vi "Agilent VNA Filter Unmeasurable Measurements.vi"(7 "Agilent VNA":T5, 8 "error in (no error)":errorcluster, 10 "Parameters to Measure":T1[](array[typedef]) {"Channel" min=1 max=99 step=1; "Parameter"."Stimulus Port" min=1 step=1; "Parameter"."Response Port" min=1 step=1}, 11 "VISA Resource Name":refnum<visa-resource-name>) -> (0 "error out":errorcluster, 1 "Removed Parameters":T1[](array[typedef]) {"Channel" min=1 max=99 step=1; "Parameter"."Stimulus Port" min=1 step=1; "Parameter"."Response Port" min=1 step=1}, 2 "Filtered Parameters to Measure":T1[](array[typedef]) {"Channel" min=1 max=99 step=1; "Parameter"."Stimulus Port" min=1 step=1; "Parameter"."Response Port" min=1 step=1}, 3 "dup VISA Resource Name":refnum<visa-resource-name>, 4 "Measurements Removed?":bool)   [LabVIEW 2011]
uses:
  tests/S Parameter/TypeDefs/SP Parameter to Measure.ctl
  tests/S Parameter/TypeDefs/SP Parameter.ctl
  tests/S Parameter/TypeDefs/SP Calibration State.ctl
  tests/S Parameter/TypeDefs/SP Measurement Format.ctl
  TypeDefs/Agilent VNA Instrument Info.ctl
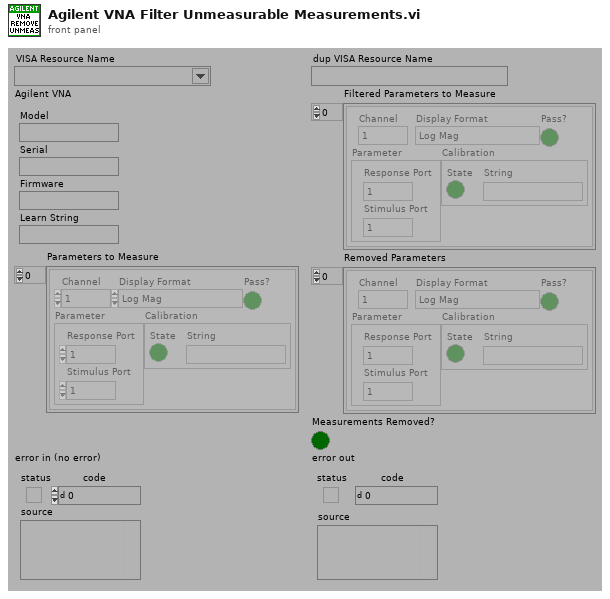
[diagram p1: front panel]
types:
  T1 = typedef "SP Parameter to Measure.ctl" = cluster{"Channel":i8, "Parameter":T2, "Calibration":T3, "Display Format":T4, "Pass?":bool}
  T2 = typedef "SP Parameter.ctl" = cluster{"Stimulus Port":i8, "Response Port":i8}
  T3 = typedef "SP Calibration State.ctl" = cluster{"State":bool, "String":string}
  T4 = typedef "SP Measurement Format.ctl" = enum32{"Log Mag", "Phase", "Delay", "Smith (R+jX)", "Polar (Re/Im)", "Linear Mag", "SWR", "Real", "Imaginary", "Smith (Lin/Phase)", "Smith (Log/Phase)", "Smith (Real/Imag)", "Smith (G+jB)", "Polar (Lin/Phase)", "Polar (Log/Phase)", "Expanded Phase", "Positive Phase", "Inverted Smith", "Unwrapped Phase", "Power Out", "Power In", "Linear Mag/Phase", "Log Mag/Phase", "Real/Imaginary"}
  T5 = typedef "Agilent VNA Instrument Info.ctl" = cluster{"Model":string, "Serial":string, "Firmware":string, "Learn String":string}
  T6 = typedef "Agilent VNA Model.ctl" = enum16{"Not Supported", "8510X", "8719X", "8720X", "8722X", "8753X", "ENA", "PNA", "Field Fox"}
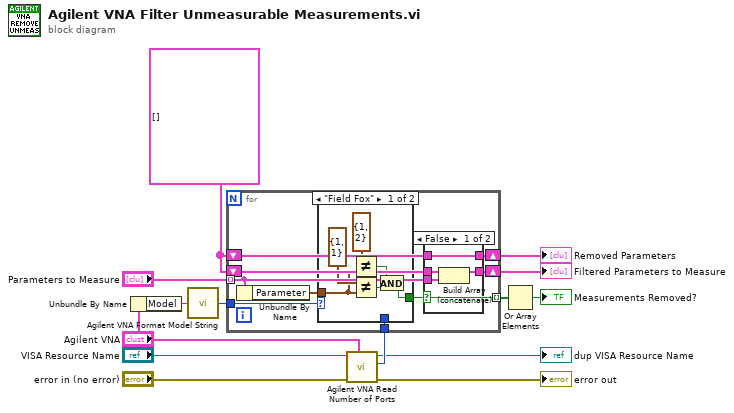
[diagram p0: block diagram]
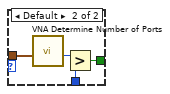
[diagram p2: hidden frame]
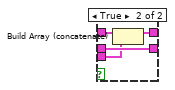
[diagram p3: hidden frame]
diagram:
  w5 = T1[] [] ("Parameters to Measure")
  n1 = Unbundle By Name("Agilent VNA") -> ("Model"=w2:string)
  n2 = call "Agilent VNA Format Model String.vi"("Model"=w2) -> ("Model"=w1:T6)
  n3 = call "Agilent VNA Read Number of Ports.vi"("Agilent VNA"="Agilent VNA", "error in (no error)"="error in (no error)", "VISA Resource Name"="VISA Resource Name") -> ("error out"=→"error out":errorcluster, "Number of Ports"=w11:i8, "dup VISA Resource Name"=→"dup VISA Resource Name":refnum<visa-resource-name>)  [unwired: 6 out]
  n4 = for {
    tunnel: "Parameters to Measure" -> [w20] mode=indexing
    shift-right: [w19] -> w8
    shift-left: w5 -> [w21]
    tunnel: w11 -> [w22]
    tunnel: [w18] -> w7 mode=indexing
    shift-right: [w16] -> w4
    shift-left: w5 -> [w17]
    tunnel: w1 -> [w15]
    n5 = Unbundle By Name(w20) -> ("Parameter"=w23:T2)
    n6 = case shown="\"Field Fox\"" w15 {
      tunnel: w23 -> [w25 w33]
      tunnel: w22 -> [_ w31]
      tunnel: [w28 w30] -> w18
      frame "Field Fox" {
        n7 = Not Equal?(x=T2 {"Stimulus Port"=1, "Response Port"=2} ("Parameter"), y=w25) -> (x != y?=w27:bool)
        n8 = Not Equal?(x=T2 {"Stimulus Port"=1, "Response Port"=1} ("Parameter"), y=w25) -> (x != y?=w29:bool)
        n9 = And(x=w27, y=w29) -> (x .and. y?=w28:bool)
      }
      frame Default {
        n10 = call "VNA Determine Number of Ports.vi"("Parameter"=w33) -> ("Number of Ports"=w32:i8)  [unwired: 10 out]
        n11 = Greater?(x=w32, y=w31) -> (0:w30:bool)
      }
    }
    n12 = case shown="False" w18 {
      tunnel: w21 -> [w37 w41]
      tunnel: w20 -> [w36 w38]
      tunnel: [w35 w41] -> w19
      tunnel: w17 -> [w34 w40]
      tunnel: [w34 w39] -> w16
      frame False {
        n13 = Build Array (concatenate)(w37, w36) -> (w35:T1[])
      }
      frame True {
        n14 = Build Array (concatenate)(w40, w38) -> (w39:T1[])
      }
    }
  }
  "Filtered Parameters to Measure" <- w8
  "Removed Parameters" <- w4
  n15 = Or Array Elements(Boolean array=w7) -> (logical OR=→"Measurements Removed?":bool)
